vi "Data Display Manager.vi"(6 "Volt Channel":T1={"Index"=[], "Chl Name"=[], "Scale"=[], "Offset"=[], "Sample Rate"=100, "Device Name"="", "Channel"=""}, 7 "Enum":T2=enum."Config Data", 8 "error in":errorcluster, 9 "Raw Data":waveform(dbl)[](array[waveform]), 11 "Data Display Choice":T3) -> (0 "error out":errorcluster, 1 "Overall Mean":dbl[](array[numeric]), 2 "Mean per Second":dbl[](array[numeric]), 3 "VI Ref":refnum<vi>)   [LabVIEW 2021]
doc: "This Vi has three functions:\nConfig Data - Reset Total Samples, Mean per Second and Overall Mean\nVolt Data - Display Data and calculate Mean per Second and Overall Mean\nDisplay Choice - Choose an appropriate displaying method and pass the chart or graph vi reference out."
uses:
  Control/Data Display Choice Enum.ctl
  Control/Data Display Manager Enum.ctl
  Control/Volt Chl.ctl
  Graph Abstract Class/Pass Ref and Receive Data -- Enum.ctl
  Graph Abstract Class/Graph Data -- cluster.ctl
  Graph Abstract Class/Display Abstract.lvclass
  Chart Class/Chart.lvclass
  Graph Class/Graph.lvclass
  <vilib>/Analysis/baseanly.llb/Mean (DBL).vi
  <vilib>/Analysis/NI_AALBase.lvlib
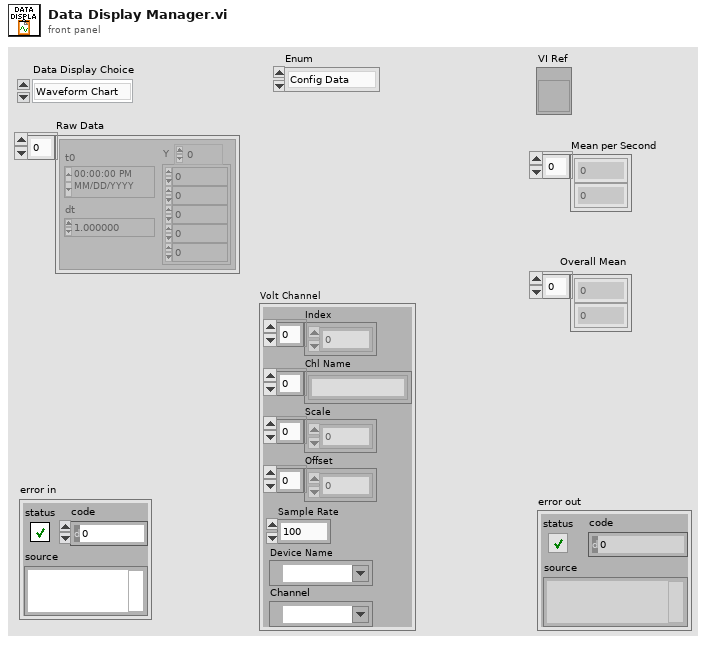
[diagram p1: front panel]
types:
  T1 = typedef "Volt Chl.ctl" = cluster{"Index":i32[], "Chl Name":string[], "Scale":dbl[], "Offset":dbl[], "Sample Rate":i32, "Device Name":tag, "Channel":tag}
  T2 = typedef "Data Display Manager Enum.ctl" = enum16{"Display Choice", "Config Data", "Volt Data"}
  T3 = typedef "Data Display Choice Enum.ctl" = enum16{"Waveform Chart", "Waveform Graph"}
  T4 = typedef "Graph Data -- cluster.ctl" = cluster{"Raw Data":waveform(dbl)[], "Volt Channel":T1}
  T5 = typedef "Pass Ref and Receive Data -- Enum.ctl" = enum16{"Initialize", "Pass Data"}
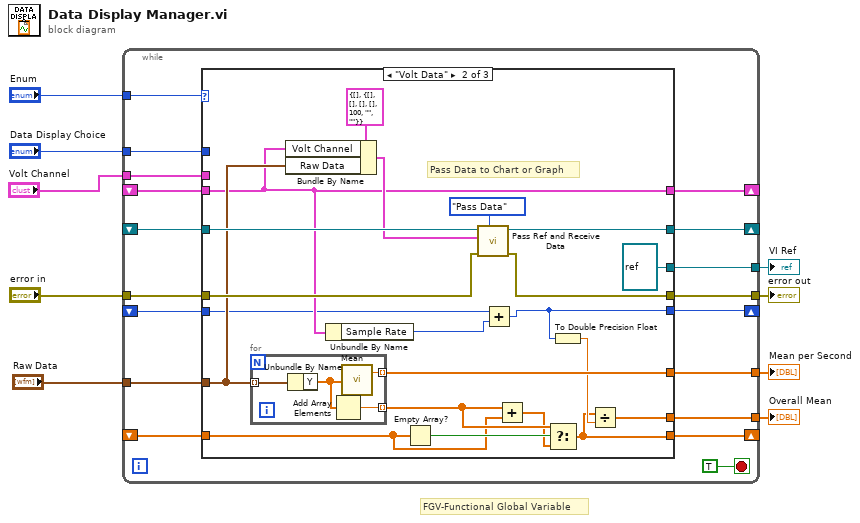
[diagram p0: block diagram]
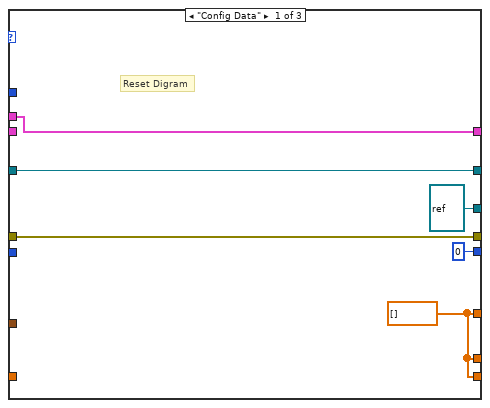
[diagram p2: hidden frame]
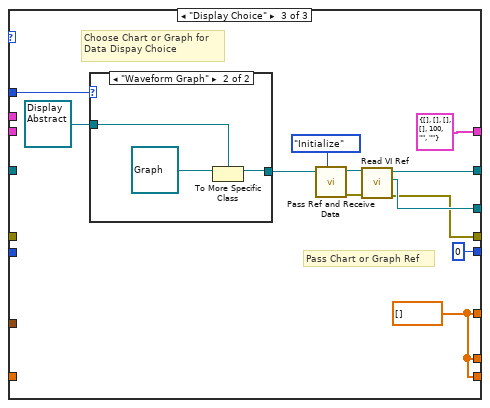
[diagram p3: hidden frame]
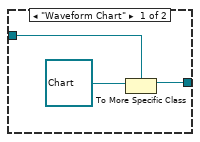
[diagram p4: hidden frame]
diagram:
  # "FGV-Functional Global Variable"
  n1 = while {
    tunnel: "Data Display Choice" -> [w27]
    shift-right: [w25] -> _
    shift-left: _ -> [w21]
    tunnel: [w23] -> w8
    tunnel: "error in" -> [w22]
    tunnel: "Enum" -> [w20]
    shift-right: [w18] -> _
    shift-left: _ -> [w19]
    tunnel: "Raw Data" -> [w17]
    tunnel: "Volt Channel" -> [w16]
    shift-right: [w15] -> _
    shift-left: _ -> [w14]
    tunnel: [w13] -> w1
    shift-right: [w12] -> _
    shift-left: _ -> [w11]
    tunnel: [w10] -> w2
    tunnel: [w24] -> w5
    stop <- TRUE stop-if-true
    n2 = case shown="\"Volt Data\"" w20 {
      tunnel: w27 -> [_ _ w69]
      tunnel: [w33 w52 w62] -> w25
      tunnel: [refnum<vi> refnum ("VI Ref") refnum<vi> refnum ("VI Ref") w67] -> w24
      tunnel: [w32 w50 w64] -> w23
      tunnel: w22 -> [w32 w49 _]
      tunnel: w21 -> [w33 w51 _]
      tunnel: w19 -> [_ w45 _]
      tunnel: [w30 w45 T1 {"Index"=[], "Chl Name"=[], "Scale"=[], "Offset"=[], "Sample Rate"=100, "Device Name"="", "Channel"=""} ("Volt Channel")] -> w18
      tunnel: w17 -> [_ w47 _]
      tunnel: w16 -> [w30 _ _]
      tunnel: [w29 w35 w60] -> w15
      tunnel: w14 -> [_ w37 _]
      tunnel: [w29 w46 w60] -> w13
      tunnel: [0 w42 0] -> w12
      tunnel: w11 -> [_ w44 _]
      tunnel: [w29 w40 w60] -> w10
      frame "Config Data" {
        w29 = dbl[] []
        # "Reset Digram"
      }
      frame "Volt Data" {
        # "Pass Data to Chart or Graph"
        n3 = for {
          tunnel: w47 -> [w58] mode=indexing
          tunnel: [w57] -> w46 mode=indexing
          tunnel: [w55] -> w38 mode=indexing
          n4 = Unbundle By Name(w58) -> ("Y"=w56:dbl[])
          n5 = Add Array Elements(numeric array=w56) -> (sum=w55:dbl)
          n6 = call-poly <vilib>:"Mean.vi"("X"=w56) -> ("mean"=w57:dbl)  [unwired: 1 out]
        }
        n7 = Bundle By Name(cluster=T4 {"Raw Data"=[], "Volt Channel"={"Index"=[], "Chl Name"=[], "Scale"=[], "Offset"=[], "Sample Rate"=100, "Device Name"="", "Channel"=""}} ("output cluster"), "Volt Channel"=w45, "Raw Data"=w47) -> (w48:T4)
        n8 = Unbundle By Name(w45) -> ("Sample Rate"=w43:i32)
        n9 = Empty Array?(array=w37) -> (empty?=w39:bool)
        n10 = call-dynamic "Pass Ref and Receive Data.vi"("Enum State"=Pass_Ref_and_Receive_Data_--_Enum."Pass Data", "error in (no error)"=w49, "Data"=w48, "Graph Manager in"=w51) -> ("error out"=w50:errorcluster, "Graph Manager out"=w52:refnum<class "Display Abstract.lvclass">)  [unwired: 6 in]
        n11 = Add(x=w44, y=w43) -> (x+y=w42:i32)
        n12 = Add(x=w38, y=w37) -> (x+y=w36:dbl[])
        n13 = Select(t=w38, s=w39, f=w36) -> (s? t:f=w35:dbl[])
        n14 = To Double Precision Float(number=w42) -> (double precision float=w41:dbl)
        n15 = Divide(x=w35, y=w41) -> (x/y=w40:dbl[])
      }
      frame "Display Choice" {
        w60 = dbl[] []
        # "Pass Chart or Graph Ref"
        # "Choose Chart or Graph for\nData Dispay Choice"
        n16 = case shown="\"Waveform Graph\"" w69 {
          tunnel: refnum<class "Display Abstract.lvclass"> refnum ("Display Abstract.lvclass") -> [w72 w75]
          tunnel: [w71 w74] -> w66
          frame "Waveform Chart" {
            n17 = To More Specific Class(target class=w72, reference=refnum<class "Chart.lvclass"> refnum ("Chart.lvclass")) -> (specific class reference=w71:refnum<class "Display Abstract.lvclass">)  [unwired: 1 in, 1 out]
          }
          frame "Waveform Graph" {
            n18 = To More Specific Class(target class=w75, reference=refnum<class "Graph.lvclass"> refnum ("Graph.lvclass")) -> (specific class reference=w74:refnum<class "Display Abstract.lvclass">)  [unwired: 1 in, 1 out]
          }
        }
        n19 = call-dynamic "Pass Ref and Receive Data.vi"("Enum State"=Pass_Ref_and_Receive_Data_--_Enum."Initialize", "Graph Manager in"=w66) -> ("error out"=w65:errorcluster, "Graph Manager out"=w63:refnum<class "Display Abstract.lvclass">)  [unwired: 8 in]
        n20 = call-dynamic "Read VI Ref.vi"("error in (no error)"=w65, "Graph Manager in"=w63) -> ("error out"=w64:errorcluster, "VI Ref"=w67:refnum<vi>, "Graph Manager out"=w62:refnum<class "Display Abstract.lvclass">)  [unwired: 7 in]
      }
    }
  }
  "error out" <- w8
  "VI Ref" <- w5
  "Overall Mean" <- w2
  "Mean per Second" <- w1
